vi "set noise_1.vi"() -> ()   [LabVIEW 2026]
uses:
  C:/Users/laserfab/Desktop/Cam-PID-LV2026/Thorlabs.MotionControl.Controls.dll
  Thorlabs.MotionControl.Controls.dll
  <vilib>/numeric/Random Number (Range) DBL.vi
  C:/Users/laserfab/Desktop/Cam-PID-LV2026/Thorlabs.MotionControl.TCube.PiezoCLI.dll
  Thorlabs.MotionControl.TCube.PiezoCLI.dll
  <vilib>/ptbypt/NI_PtbyPt.lvlib
panel:
  out "Tension Y":dbl=30.0
  out "Tension X":dbl=20.0
  in  "Choix Tension Y":T1(ring)=enum."30V"
  in  "Choix Tension X":T1(ring)=enum."20V"
  in  "piezo start":bool
  in  "stop":bool=TRUE
  out "Graphe Y":cluster{"number":dbl, dbl}(graph)={"number"=30.0, 50.0}
  out "Graphe X":cluster{"number":dbl, dbl}(graph)={"number"=20.0, 50.0}
  in  "Model":T2(ring)=enum."sinus"
  out "GetOutputVoltage Y":dbl=29.9844355601672
  out "GetOutputVoltage X":dbl=19.968260750145
  in  "TCubePiezoControl 4":refnum<k24>(container)
  in  "SerialNumber Y":string="81844665"
  out "CreateDevice Y":bool=TRUE
  out "CloseDevice Y":bool=TRUE
  in  "TCubePiezoControl 3":refnum<k24>(container)
  in  "SerialNumber X":string="81844656"
  out "CreateDevice X":bool=TRUE
  out "CloseDevice X":bool=TRUE
  in  "Commande onglets":enum32{"initial", "sin", "gauss"}(tab)=enum."sin"
  in  "frequency sin X":dbl=25.0 caption="fréquence" format="%0.2f"
  in  "delta sin X":dbl=1000.0
  out "dt sin X":dbl=0.636
  in  "frequency sin Y":dbl=10.0 caption="fréquence Y" format="%0.2f"
  in  "delta sin Y":dbl=1000.0
  out "dt sin Y":dbl=0.636
  in  "dephasage":bool
  in  "-x":dbl=-1.0 format="%#_13g"
  in  "Amplitude X":dbl=50.0 format="%#_13g"
  in  "Amplitude Y":dbl=50.0 format="%#_13g"
  in  "amplitute target Y":dbl=50.0 format="%#_13g"
  in  "amplitute target X":dbl=20.0 format="%#_13g"
  in  "Ecart type X":dbl=0.35 caption="écart-type" format="%0.2f"
  # "Change Serial Number"
  # "Change Serial Number"
  # "sinus\nX"
  # "sinus\nY"
  # "Gaussien Y"
  # "Gaussien X"
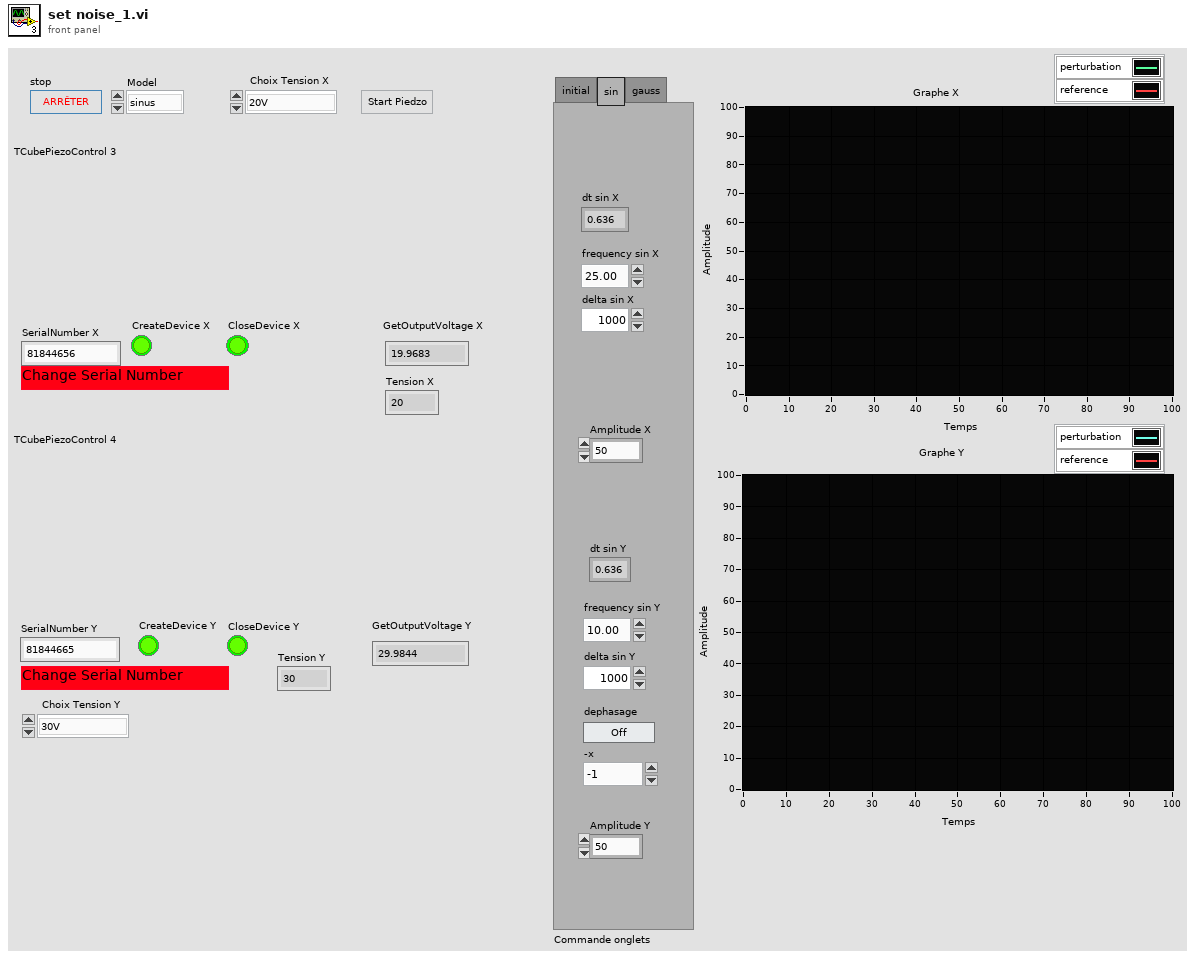
[diagram p1: front panel]
types:
  T1 = enum16{"0V", "10V", "20V", "30V", "40V", "50V", "60V", "70V", "80V", "90V", "100V"}
  T2 = enum16{"initial", "aléatoire", "gaussien", "sinus"}
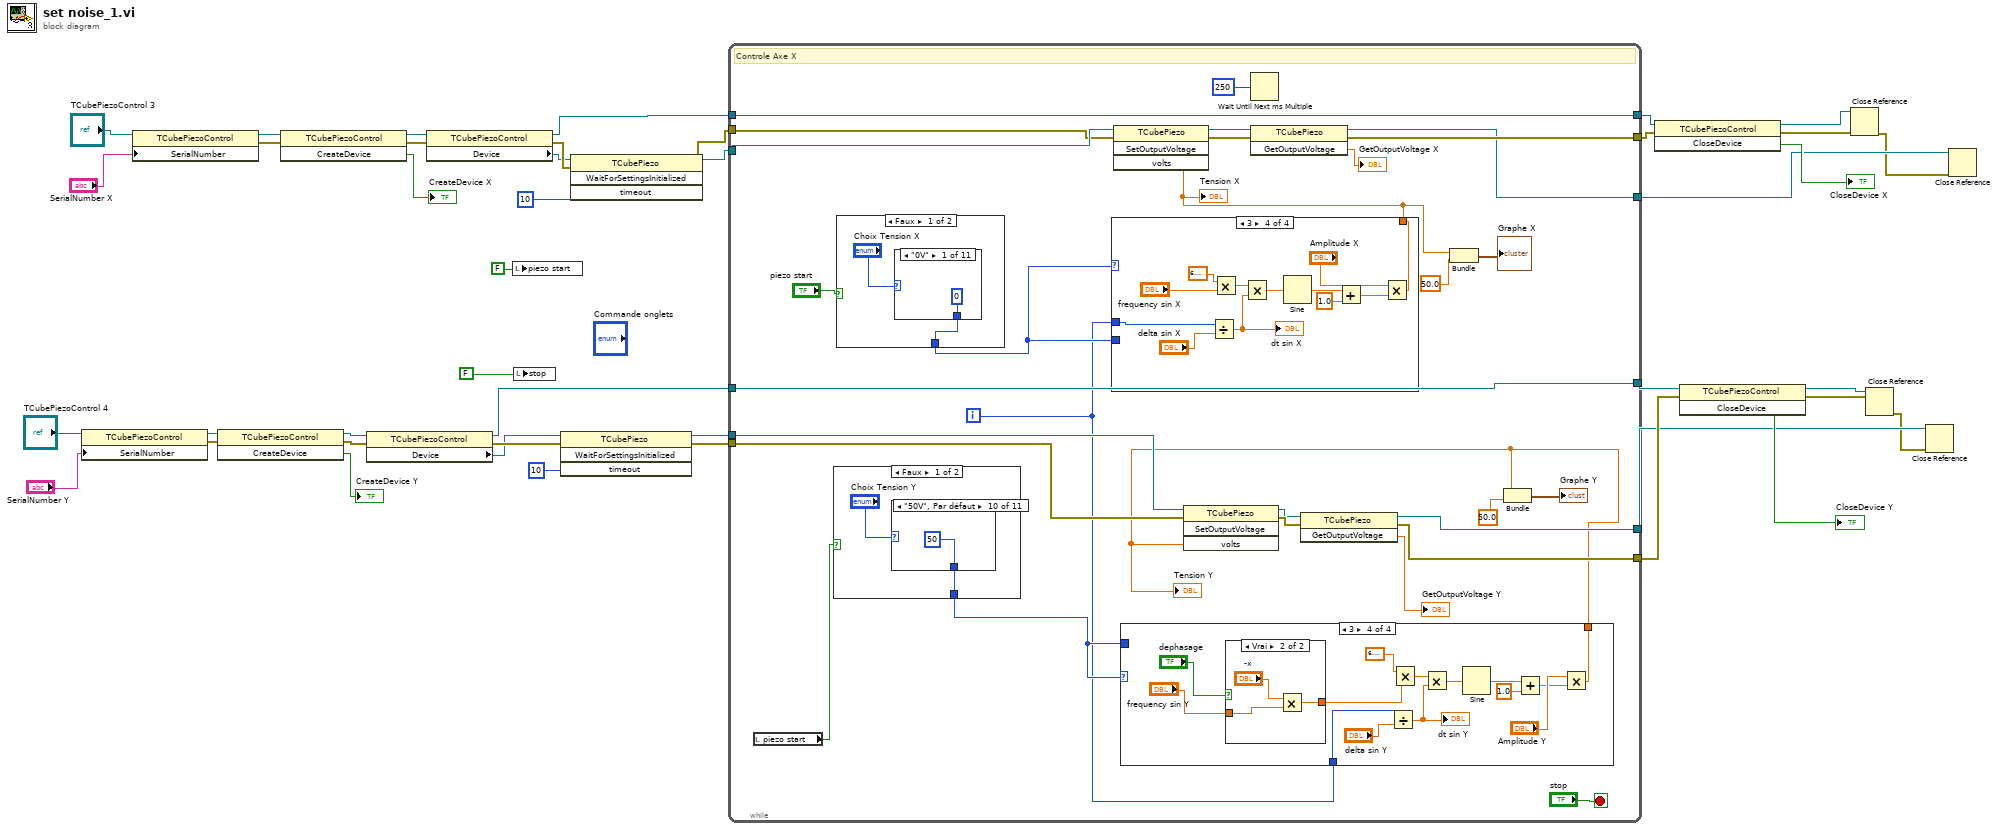
[diagram p0: block diagram]
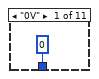
[diagram p2: hidden frame]
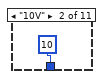
[diagram p3: hidden frame]
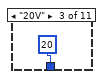
[diagram p4: hidden frame]
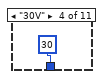
[diagram p5: hidden frame]
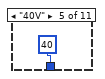
[diagram p6: hidden frame]
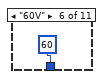
[diagram p7: hidden frame]
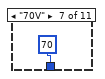
[diagram p8: hidden frame]
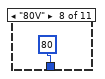
[diagram p9: hidden frame]
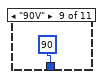
[diagram p10: hidden frame]
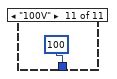
[diagram p11: hidden frame]
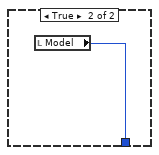
[diagram p12: hidden frame]
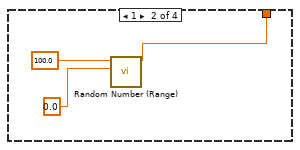
[diagram p14: hidden frame]
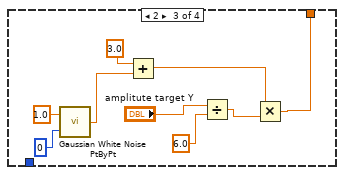
[diagram p15: hidden frame]
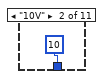
[diagram p17: hidden frame]
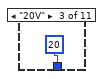
[diagram p18: hidden frame]
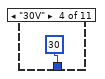
[diagram p19: hidden frame]
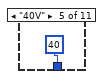
[diagram p20: hidden frame]
diagram:
  n1 = property on="Nœud de propriété" class="TCubePiezoControl"(reference="TCubePiezoControl 4", "SerialNumber"="SerialNumber Y") -> (reference out=w18:refnum<k24>, error out=w19:errorcluster)  [unwired: 1 in]
  n2 = property on="Nœud de propriété" class="TCubePiezoControl"(reference="TCubePiezoControl 3", "SerialNumber"="SerialNumber X") -> (reference out=w31:refnum<k24>, error out=w32:errorcluster)  [unwired: 1 in]
  n3 = invoke on="Nœud de méthode" class="TCubePiezoControl" method="CreateDevice"(reference=w18, error in=w19) -> (reference out=w21:refnum<k24>, error out=w20:errorcluster, "CreateDevice"=→"CreateDevice Y":bool)  [unwired: 1 in]
  n4 = invoke on="Nœud de méthode" class="TCubePiezoControl" method="CreateDevice"(reference=w31, error in=w32) -> (reference out=w34:refnum<k24>, error out=w33:errorcluster, "CreateDevice"=→"CreateDevice X":bool)  [unwired: 1 in]
  n5 = property on="Nœud de propriété" class="TCubePiezoControl"(reference=w21, error in=w20) -> (reference out=w12:refnum<k24>, error out=w24:errorcluster, "Device"=w23:refnum<k24>)
  n6 = property on="Nœud de propriété" class="TCubePiezoControl"(reference=w34, error in=w33) -> (reference out=w36:refnum<k24>, error out=w39:errorcluster, "Device"=w38:refnum<k24>)
  n7 = local write "piezo start"(FALSE ("piezo start")) -> ()
  n8 = local write "stop"(FALSE ("stop")) -> ()
  n9 = invoke on="Nœud de méthode" class="TCubePiezo" method="WaitForSettingsInitialized"(reference=w23, error in=w24, "timeout"=10) -> (reference out=w11:refnum<k24>, error out=w13:errorcluster)  [unwired: 1 in, 2 out]
  n10 = invoke on="Nœud de méthode" class="TCubePiezo" method="WaitForSettingsInitialized"(reference=w38, error in=w39, "timeout"=10) -> (reference out=w41:refnum<k24>, error out=w42:errorcluster)  [unwired: 1 in, 2 out]
  n11 = while {
    tunnel: w36 -> [w71]
    tunnel: [w71] -> w26
    tunnel: [w70] -> w37
    tunnel: w41 -> [w67]
    tunnel: w42 -> [w66]
    tunnel: w13 -> [w50]
    tunnel: [w49] -> w5
    tunnel: w12 -> [w49]
    tunnel: w11 -> [w48]
    tunnel: [w47] -> w4
    tunnel: [w46] -> w8
    tunnel: [w45] -> w3
    i -> [w43]
    stop <- "stop" stop-if-true
    # "Controle Axe X"
    n12 = local read "piezo start"() -> (w57:bool)
    n13 = case shown="Faux" w57 {
      tunnel: [w73 w85] -> w56
      frame False {
        n14 = case shown="\"50V\", Par défaut" "Choix Tension Y" {
          tunnel: [0 10 20 30 40 60 70 80 90 50 100] -> w73
          frame "0V" {
          }
          frame "10V" {
          }
          frame "20V" {
          }
          frame "30V" {
          }
          frame "40V" {
          }
          frame "60V" {
          }
          frame "70V" {
          }
          frame "80V" {
          }
          frame "90V" {
          }
          frame "50V", Default {
          }
          frame "100V" {
          }
        }
      }
      frame True {
        n15 = local read "Model"() -> (w85:T2)
      }
    }
    n16 = case shown="Faux" "piezo start" {
      tunnel: [w118 "Model"] -> w62
      frame False {
        n17 = case shown="\"0V\"" "Choix Tension X" {
          tunnel: [0 10 20 30 40 60 70 80 90 50 100] -> w118
          frame "0V" {
          }
          frame "10V" {
          }
          frame "20V" {
          }
          frame "30V" {
          }
          frame "40V" {
          }
          frame "60V" {
          }
          frame "70V" {
          }
          frame "80V" {
          }
          frame "90V" {
          }
          frame "50V", Default {
          }
          frame "100V" {
          }
        }
      }
      frame True {
      }
    }
    n18 = case shown="3" w62 {
      tunnel: [w131 w133 w135 w150] -> w60
      tunnel: w43 -> [_ _ _ w151]
      tunnel: w62 -> [w131 _ _ _]
      frame 0, Default {
      }
      frame 1 {
        n19 = call-poly <vilib>:"Random Number (Range).vi"("lower bound (0)"=0.0, "upper bound (100)"=100.0) -> ("number"=w133:dbl)  [unwired: 9 in]
      }
      frame 2 {
        n20 = disable-structure shown="Activé" {
          disable-tunnel: [w136 w145] -> w135
          frame Disabled {
            n21 = call <vilib>:"Gaussian White Noise PtByPt.vi"("seed"=0, "standard deviation"=1.0) -> ("Gaussian white noise"=w142:dbl)  [unwired: 1 in]
            n22 = Add(x=3.0, y=w142) -> (x+y=w141:dbl)
            n23 = Divide(x="amplitute target X", y=6.0) -> (x/y=w139:dbl)
            n24 = Multiply(x=w141, y=w139) -> (x*y=w136:dbl)
          }
          frame Enabled {
            w146 = 50.0 ("y")
            n25 = call <vilib>:"Gaussian White Noise PtByPt.vi"("standard deviation"="Ecart type X") -> ("Gaussian white noise"=w148:dbl)  [unwired: 2 in]
            n26 = Multiply(x=w148, y=w146) -> (x*y=w147:dbl)
            n27 = Add(x=w147, y=w146) -> (x+y=w145:dbl)
          }
        }
      }
      frame 3 {
        n28 = Divide(x=w151, y="delta sin X") -> (x/y=w158:dbl)
        "dt sin X" <- w158
        n29 = Multiply(x=6.283185307179586, y="frequency sin X") -> (x*y=w160:dbl)
        n30 = Multiply(x=w160, y=w158) -> (x*y=w157:dbl)
        n31 = Sine(x=w157) -> (sin(x)=w156:dbl)
        n32 = Add(x=w156, y=1.0) -> (x+y=w155:dbl)
        n33 = Multiply(x="Amplitude X", y=w155) -> (x*y=w150:dbl)
      }
    }
    "Tension X" <- w60
    n34 = invoke on="Nœud de méthode" class="TCubePiezo" method="SetOutputVoltage"(reference=w67, error in=w66, "volts"=w60) -> (reference out=w65:refnum<k24>, error out=w64:errorcluster)  [unwired: 1 in, 2 out]
    n35 = case shown="3" w56 {
      tunnel: [w86 w89 w90 w103] -> w44
      tunnel: w43 -> [_ _ _ w102]
      tunnel: w56 -> [w86 _ _ _]
      frame 0, Default {
      }
      frame 1 {
        n36 = call-poly <vilib>:"Random Number (Range).vi"("lower bound (0)"=0.0, "upper bound (100)"=100.0) -> ("number"=w89:dbl)  [unwired: 9 in]
      }
      frame 2 {
        n37 = call <vilib>:"Gaussian White Noise PtByPt.vi"("seed"=0, "standard deviation"=1.0) -> ("Gaussian white noise"=w96:dbl)  [unwired: 1 in]
        n38 = Add(x=3.0, y=w96) -> (x+y=w95:dbl)
        n39 = Divide(x="amplitute target Y", y=6.0) -> (x/y=w93:dbl)
        n40 = Multiply(x=w95, y=w93) -> (x*y=w90:dbl)
      }
      frame 3 {
        n41 = case shown="Vrai" "dephasage" {
          tunnel: "frequency sin Y" -> [w113 w116]
          tunnel: [w113 w114] -> w99
          frame False {
          }
          frame True {
            n42 = Multiply(x="-x", y=w116) -> (x*y=w114:dbl)
          }
        }
        n43 = Divide(x=w102, y="delta sin Y") -> (x/y=w106:dbl)
        "dt sin Y" <- w106
        n44 = Multiply(x=6.283185307179586, y=w99) -> (x*y=w104:dbl)
        n45 = Multiply(x=w104, y=w106) -> (x*y=w107:dbl)
        n46 = Sine(x=w107) -> (sin(x)=w108:dbl)
        n47 = Add(x=w108, y=1.0) -> (x+y=w109:dbl)
        n48 = Multiply(x="Amplitude Y", y=w109) -> (x*y=w103:dbl)
      }
    }
    "Tension Y" <- w44
    n49 = invoke on="Nœud de méthode" class="TCubePiezo" method="SetOutputVoltage"(reference=w48, error in=w50, "volts"=w44) -> (reference out=w53:refnum<k24>, error out=w54:errorcluster)  [unwired: 1 in, 2 out]
    n50 = Wait Until Next ms Multiple(millisecond multiple=u32 250 ("n millisecondes")) -> ()  [unwired: 1 out]
    n51 = invoke on="Nœud de méthode" class="TCubePiezo" method="GetOutputVoltage"(reference=w65, error in=w64) -> (reference out=w45:refnum<k24>, error out=w70:errorcluster, "GetOutputVoltage"=→"GetOutputVoltage X":dbl)  [unwired: 1 in]
    n52 = invoke on="Nœud de méthode" class="TCubePiezo" method="GetOutputVoltage"(reference=w53, error in=w54) -> (reference out=w47:refnum<k24>, error out=w46:errorcluster, "GetOutputVoltage"=→"GetOutputVoltage Y":dbl)  [unwired: 1 in]
    n53 = Bundle("number"=w60, 50.0) -> (→"Graphe X":cluster{"number":dbl, dbl})  [unwired: 1 in]
    n54 = Bundle("number"=w44, 50.0) -> (→"Graphe Y":cluster{"number":dbl, dbl})  [unwired: 1 in]
  }
  n55 = invoke on="Nœud de méthode" class="TCubePiezoControl" method="CloseDevice"(reference=w26, error in=w37) -> (reference out=w9:refnum<k24>, error out=w6:errorcluster, "CloseDevice"=→"CloseDevice X":bool)  [unwired: 1 in]
  n56 = invoke on="Nœud de méthode" class="TCubePiezoControl" method="CloseDevice"(reference=w5, error in=w8) -> (reference out=w10:refnum<k24>, error out=w7:errorcluster, "CloseDevice"=→"CloseDevice Y":bool)  [unwired: 1 in]
  n57 = Close Reference(reference=w9, error in (no error)=w6) -> (error out=w2:errorcluster)
  n58 = Close Reference(reference=w10, error in (no error)=w7) -> (error out=w1:errorcluster)
  n59 = Close Reference(reference=w4, error in (no error)=w1) -> ()  [unwired: 1 out]
  n60 = Close Reference(reference=w3, error in (no error)=w2) -> ()  [unwired: 1 out]
